vi "Bundle Script_Properties Rearrange.vi"(8 "error in":errorcluster, 10 "Property Array":T2(array[cluster]), 11 "Affected Items":T1) -> (0 "error out":errorcluster, 2 "Objects":refnum<vi>[](array[refnum]))   [LabVIEW 2023]
doc: "Tag tree tags as nput, as these contain the original indices, which are used for reordering the wires and labels of the bundle or unbundle by name structures"
uses:
  top/BundleMagic.ctl
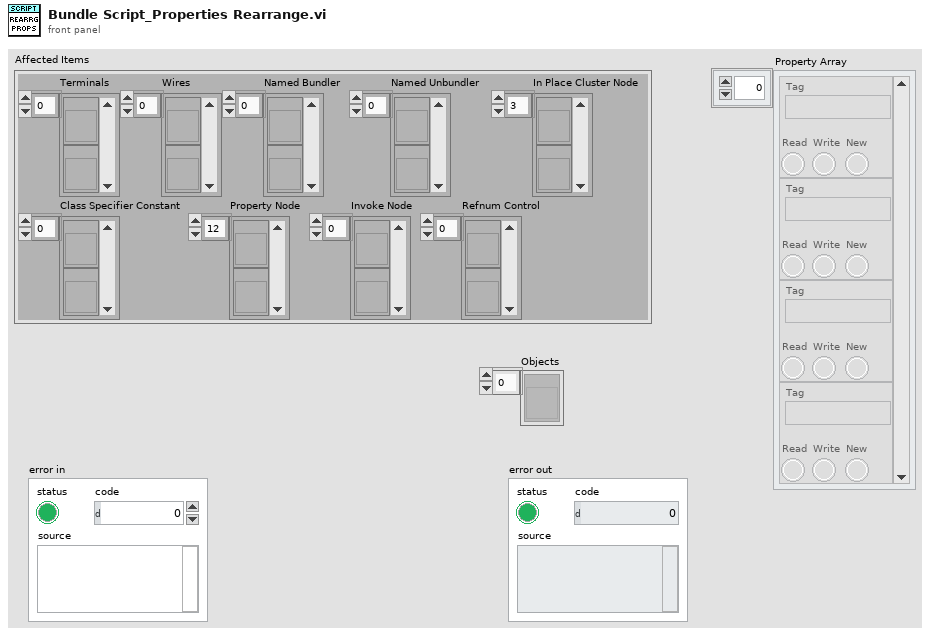
[diagram p1: front panel]
types:
  T1 = typedef "BundleMagic.ctl" = cluster{"Terminals":refnum<vi>[], "Wires":refnum<vi>[], "Named Bundler":refnum<vi>[], "Named Unbundler":refnum<vi>[], "In Place Cluster Node":refnum<vi>[], "Class Specifier Constant":refnum<vi>[], "Property Node":refnum<vi>[], "Invoke Node":refnum<vi>[], "Refnum Control":refnum<vi>[]}
  T2 = cluster{"Tag":string, "Read":bool, "Write":bool, "New":bool}[]
  T3 = cluster{"Index":u16, "Property Type":enum16{"Unknown", "Base", "Scripting", "Private", "Deprecated", "None", "Divider"}, "ID String":string, "Dotted ID String":string, "Class":string, "Parent":string, "Display name full":string, "Display name short":string, "Parents Array":string[], "Indent":u16}
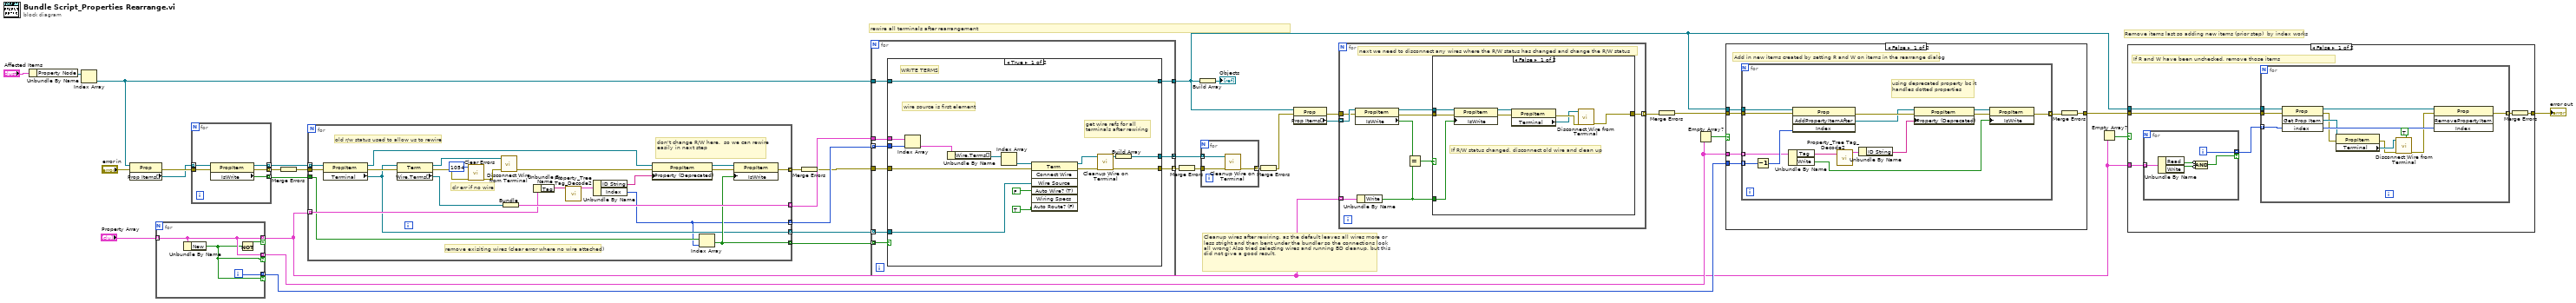
[diagram p0: block diagram]
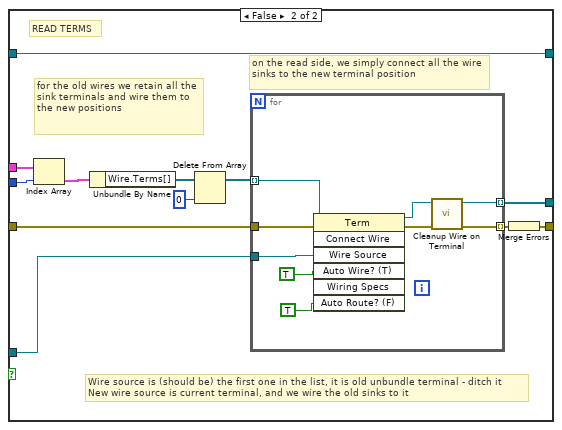
[diagram p4: hidden frame]
diagram:
  # "Remove items last so adding new items (prior step)  by index works"
  # "rewire all terminals after rearrangement"
  # "Cleanup wires after rewiring, as the default leaves all wires more or less stright and then bent under the bundler so the connections look all wrong! Also tried selecting wires and running BD cleanup, but this did not give a good result."
  n1 = Unbundle By Name("Affected Items") -> ("Property Node"=w33:refnum<vi>[])
  n2 = Index Array(array=w33) -> (element=w27:refnum<vi>)  [unwired: 1 in]
  n3 = property class="Prop"(reference=w27, error in="error in") -> (error out=w25:errorcluster, "Prop Items[]"=w23:refnum<vi>[])  [unwired: 1 out]
  n4 = for {
    tunnel: "Property Array" -> [w39] mode=indexing
    tunnel: [w39] -> w8 mode=indexing if=w36
    tunnel: [w39] -> w12 mode=indexing if=w37
    tunnel: [w38] -> w13 mode=indexing if=w37
    i -> [w38]
    n5 = Unbundle By Name(w39) -> ("New"=w37:bool)
    n6 = Not(x=w37) -> (.not. x?=w36:bool)
  }
  n7 = for {
    tunnel: w25 -> [w44]
    tunnel: [w43] -> w26 mode=indexing
    tunnel: w23 -> [w42] mode=indexing
    tunnel: [w41] -> w22 mode=indexing
    tunnel: [w40] -> w21 mode=indexing
    n8 = property class="PropItem"(reference=w42, error in=w44) -> (reference out=w41:refnum<vi>, error out=w43:errorcluster, "IsWrite"=w40:bool)
  }
  n9 = Merge Errors(w26) -> (w24:errorcluster)
  n10 = for {
    tunnel: [w65] -> w35 mode=indexing
    tunnel: w24 -> [w59]
    tunnel: [w61] -> w34 mode=indexing
    tunnel: w8 -> [w63] mode=indexing
    tunnel: [w50] -> w30 mode=indexing
    tunnel: [w56] -> w19 mode=indexing
    tunnel: w22 -> [w60] mode=indexing
    tunnel: w21 -> [w62]
    tunnel: [w58] -> w20 mode=indexing
    # "clr err if no wire"
    # "don't change R/W here,  so we can rewire easily in next step"
    # "remove exisiting wires (clear error where no wire attached)"
    # "old r/w status used to allow us to rewire"
    n11 = property class="PropItem"(reference=w60, error in=w59) -> (reference out=w49:refnum<vi>, error out=w64:errorcluster, "Terminal"=w56:refnum<vi>)
    n12 = property class="Term"(reference=w56, error in=w64) -> (reference out=w55:refnum<vi>, error out=w57:errorcluster, "Wire.Terms[]"=w66:refnum<vi>[])
    n13 = call <vilib>:"Clear Errors.vi"("error in (no error)"=w57, "specific error code to clear (0: all)"=1054) -> ("error out"=w54:errorcluster)  [unwired: 4 in, 1 out]
    n14 = call "Disconnect Wire from Terminal.vi"("error in"=w54, "Terminal in"=w55) -> ("error out"=w48:errorcluster)  [unwired: 5 in, 4 out]
    n15 = Bundle("Wire.Terms[]"=w66) -> (w65:cluster{"Wire.Terms[]":refnum<vi>[]})  [unwired: 1 in]
    n16 = Unbundle By Name(w63) -> ("Tag"=w51:string)
    n17 = call "Property_Tree Tag_Decode2.vi"("Tag In"=w51) -> ("TagData"=w52:T3)  [unwired: 10 in]
    n18 = Unbundle By Name(w52) -> ("ID String"=w47:string, "Index"=w50:u16)
    n19 = property class="PropItem"(reference=w49, error in=w48, "Property (Deprecated)"=w47) -> (reference out=w45:refnum<vi>, error out=w46:errorcluster)
    n20 = Index Array(array=w62, index=w50) -> (element=w58:bool)
    n21 = property class="PropItem"(reference=w45, error in=w46, "IsWrite"=w58) -> (error out=w61:errorcluster)  [unwired: 1 out]
  }
  n22 = Merge Errors(w34) -> (w3:errorcluster)
  n23 = for {
    tunnel: w35 -> [w75]
    tunnel: w30 -> [w72] mode=indexing
    tunnel: w19 -> [w69] mode=indexing
    tunnel: w27 -> [w73]
    tunnel: [w70] -> w9
    tunnel: w3 -> [w74]
    tunnel: [w71] -> w29 mode=indexing
    tunnel: w20 -> [w68] mode=indexing
    tunnel: [w67] -> w10 mode=concatenating
    n24 = case shown="True" w68 {
      tunnel: w74 -> [w90 w101]
      tunnel: w75 -> [w89 w102]
      tunnel: w73 -> [w87 w98]
      tunnel: w72 -> [w88 w100]
      tunnel: [w78 w91] -> w71
      tunnel: [w87 w98] -> w70
      tunnel: w69 -> [w83 w97]
      tunnel: [w76 w92] -> w67
      frame True {
        # "get wire refs for all terminals after rewiring"
        # "WRITE TERMS"
        # "wire source is first element"
        n25 = Index Array(array=w89, index=w88) -> (element=w86:cluster{"Wire.Terms[]":refnum<vi>[]})
        n26 = Unbundle By Name(w86) -> ("Wire.Terms[]"=w85:refnum<vi>[])
        n27 = Index Array(array=w85) -> (element=w84:refnum<vi>)  [unwired: 1 in]
        n28 = invoke class="Term" method="Connect Wire"(reference=w84, error in=w90, "Wire Source"=w83, "Auto Wire? (T)"=FALSE, "Auto Route? (F)"=TRUE) -> (reference out=w80:refnum<vi>, error out=w79:errorcluster)  [unwired: 2 in, 5 out]
        n29 = call "Cleanup Wire on Terminal.vi"("error in"=w79, "Terminal in"=w80) -> ("error out"=w78:errorcluster, "Terminal Out"=w77:refnum<vi>)  [unwired: 7 in, 1 out]
        n30 = Build Array(w77) -> (w76:refnum<vi>[])
      }
      frame False {
        # "READ TERMS"
        # "for the old wires we retain all the sink terminals and wire them to the new positions"
        # "Wire source is (should be) the first one in the list, it is old unbundle terminal - ditch it\nNew wire source is current terminal, and we wire the old sinks to it"
        # "on the read side, we simply connect all the wire sinks to the new terminal position"
        n31 = Index Array(array=w102, index=w100) -> (element=w95:cluster{"Wire.Terms[]":refnum<vi>[]})
        n32 = Unbundle By Name(w95) -> ("Wire.Terms[]"=w96:refnum<vi>[])
        n33 = Delete From Array(array=w96, index=0) -> (array with subset deleted=w93:refnum<vi>[])  [unwired: 1 in, 1 out]
        n34 = for {
          tunnel: w101 -> [w111]
          tunnel: w93 -> [w104] mode=indexing
          tunnel: w97 -> [w109]
          tunnel: [w105] -> w99 mode=indexing
          tunnel: [w103] -> w92 mode=indexing
          n35 = invoke class="Term" method="Connect Wire"(reference=w104, error in=w111, "Wire Source"=w109, "Auto Wire? (T)"=TRUE ("Auto Route? (F)"), "Auto Route? (F)"=TRUE) -> (reference out=w107:refnum<vi>, error out=w106:errorcluster)  [unwired: 2 in, 5 out]
          n36 = call "Cleanup Wire on Terminal.vi"("error in"=w106, "Terminal in"=w107) -> ("error out"=w105:errorcluster, "Terminal Out"=w103:refnum<vi>)  [unwired: 7 in, 1 out]
        }
        n37 = Merge Errors(w99) -> (w91:errorcluster)
      }
    }
  }
  n38 = Merge Errors(w29) -> (w2:errorcluster)
  n39 = Build Array(w9) -> (→"Objects":refnum<vi>[])
  n40 = for {
    tunnel: w10 -> [w113] mode=indexing
    tunnel: w2 -> [w114]
    tunnel: [w112] -> w15 mode=indexing
    n41 = call "Cleanup Wire on Terminal.vi"("error in"=w114, "Terminal in"=w113) -> ("error out"=w112:errorcluster)  [unwired: 7 in, 2 out]
  }
  n42 = Merge Errors(w15) -> (w1:errorcluster)
  n43 = property class="Prop"(reference=w9, error in=w1) -> (error out=w17:errorcluster, "Prop Items[]"=w18:refnum<vi>[])  [unwired: 1 out]
  n44 = for {
    tunnel: w8 -> [w123] mode=indexing
    tunnel: w18 -> [w119] mode=indexing
    tunnel: w17 -> [w117]
    tunnel: [w120] -> w16 mode=indexing
    # "next we need to disconnect any wires where the R/W status has changed and change the R/W status"
    n45 = property class="PropItem"(reference=w119, error in=w117) -> (reference out=w118:refnum<vi>, error out=w116:errorcluster, "IsWrite"=w115:bool)
    n46 = Unbundle By Name(w123) -> ("Write"=w121:bool)
    n47 = Equal?(x=w115, y=w121) -> (x = y?=w122:bool)
    n48 = case shown="False" w122 {
      tunnel: w121 -> [w131 _]
      tunnel: w116 -> [w130 w132]
      tunnel: [w124 w132] -> w120
      tunnel: w118 -> [w129 _]
      frame False {
        # "If R/W status changed, disconnect old wire and clean up"
        n49 = property class="PropItem"(reference=w129, error in=w130, "IsWrite"=w131) -> (reference out=w128:refnum<vi>, error out=w127:errorcluster)
        n50 = property class="PropItem"(reference=w128, error in=w127) -> (error out=w126:errorcluster, "Terminal"=w125:refnum<vi>)  [unwired: 1 out]
        n51 = call "Disconnect Wire from Terminal.vi"("error in"=w126, "Terminal in"=w125) -> ("error out"=w124:errorcluster)  [unwired: 5 in, 4 out]
      }
      frame True {
      }
    }
  }
  n52 = Merge Errors(w16) -> (w6:errorcluster)
  n53 = Empty Array?(array=w12) -> (empty?=w11:bool)
  n54 = case shown="False" w11 {
    tunnel: w9 -> [w138 _]
    tunnel: w12 -> [w137 _]
    tunnel: w13 -> [w136 _]
    tunnel: w6 -> [w134 w153]
    tunnel: [w133 w153] -> w5
    frame False {
      # "Add in new items created by setting R and W on items in the rearrange dialog"
      n55 = for {
        tunnel: w138 -> [w152]
        tunnel: w137 -> [w149] mode=indexing
        tunnel: w136 -> [w151] mode=indexing
        tunnel: [w148] -> w135 mode=indexing
        tunnel: w134 -> [w146]
        # "using deprecated property bc it handles dotted properties"
        n56 = Decrement(x=w151) -> (x-1=w150:i32)
        n57 = Unbundle By Name(w149) -> ("Tag"=w144:string, "Write"=w147:bool)
        n58 = invoke class="Prop" method="AddPropertyItemAfter"(reference=w152, error in=w146, "Index"=w150) -> (error out=w143:errorcluster, "AddPropertyItemBefore"=w142:refnum<vi>)  [unwired: 1 in, 2 out]
        n59 = call "Property_Tree Tag_Decode2.vi"("Tag In"=w144) -> ("TagData"=w145:T3)  [unwired: 10 in]
        n60 = Unbundle By Name(w145) -> ("ID String"=w139:string)
        n61 = property class="PropItem"(reference=w142, error in=w143, "Property (Deprecated)"=w139) -> (reference out=w141:refnum<vi>, error out=w140:errorcluster)
        n62 = property class="PropItem"(reference=w141, error in=w140, "IsWrite"=w147) -> (error out=w148:errorcluster)  [unwired: 1 out]
      }
      n63 = Merge Errors(w135) -> (w133:errorcluster)
    }
    frame True {
    }
  }
  n64 = Empty Array?(array=w8) -> (empty?=w7:bool)
  n65 = case shown="False" w7 {
    tunnel: w9 -> [w159 _]
    tunnel: w8 -> [w156 _]
    tunnel: w5 -> [w155 w176]
    tunnel: [w154 w176] -> w4
    frame False {
      # "If R and W have been unchecked, remove those items"
      n66 = for {
        tunnel: w156 -> [w164] mode=indexing
        tunnel: [w161] -> w158 mode=indexing if=w160
        i -> [w161]
        n67 = Unbundle By Name(w164) -> ("Read"=w163:bool, "Write"=w162:bool)
        n68 = Compound Arithmetic op=AND(invert w163, invert w162) -> (w160:bool)
      }
      n69 = for {
        tunnel: w159 -> [w174]
        tunnel: w158 -> [w173] mode=indexing
        tunnel: [w175] -> w157 mode=indexing
        tunnel: w155 -> [w165]
        n70 = invoke class="Prop" method="Get Prop Item"(reference=w174, error in=w165, "index"=w173) -> (reference out=w168:refnum<vi>, error out=w170:errorcluster, "Get Prop Item"=w172:refnum<vi>)  [unwired: 1 in, 1 out]
        n71 = property class="PropItem"(reference=w172, error in=w170) -> (error out=w169:errorcluster, "Terminal"=w171:refnum<vi>)  [unwired: 1 out]
        n72 = call "Disconnect Wire from Terminal.vi"("Remove Loose Ends"=TRUE, "error in"=w169, "Terminal in"=w171) -> ("error out"=w167:errorcluster)  [unwired: 4 in, 4 out]
        n73 = invoke class="Prop" method="RemovePropertyItem"(reference=w168, error in=w167, "Index"=w173) -> (error out=w175:errorcluster)  [unwired: 1 in, 3 out]
      }
      n74 = Merge Errors(w157) -> (w154:errorcluster)
    }
    frame True {
    }
  }
  "error out" <- w4
